vi "DMM Control.vi"(8 "error in (no error)":errorcluster, 10 "JSONCluster":T1 {"DMMVoltageFaultUpperLimit" format="%#_6p"}, 11 "IVI Refnum in":refnum<k15>) -> (0 "error out":errorcluster, 3 "IVI Refnum out":refnum<k15>)   [LabVIEW 2019, in "SupportVIs.lvlib"]
uses:
  SupportVIs.lvlib
  JSONCluster.ctl
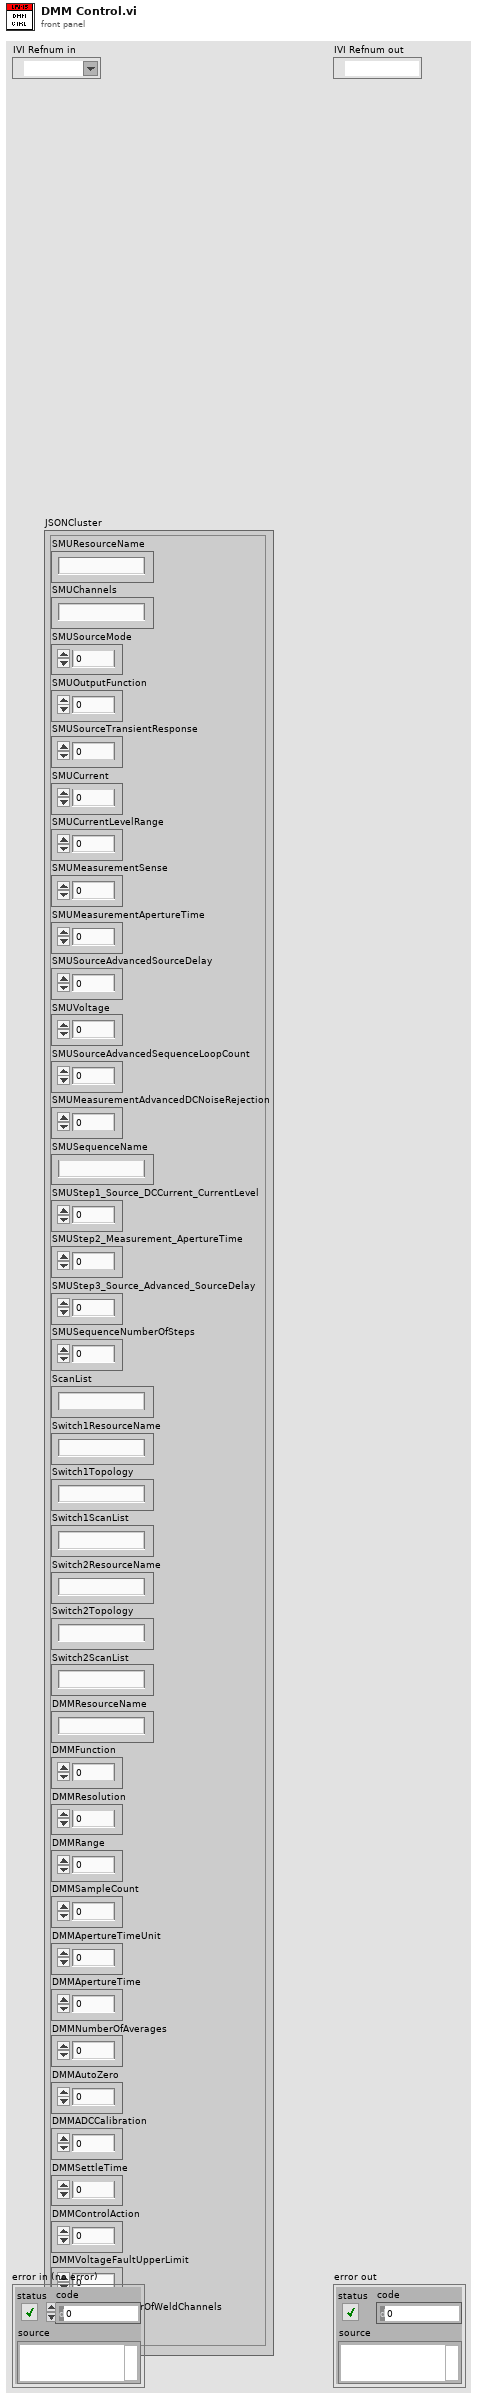
[diagram p1: front panel]
types:
  T1 = typedef "JSONCluster.ctl" = cluster{"SMUResourceName":string, "SMUChannels":string, "SMUSourceMode":i32, "SMUOutputFunction":i32, "SMUSourceTransientResponse":i32, "SMUCurrent":dbl, "SMUCurrentLevelRange":dbl, "SMUMeasurementSense":i32, "SMUMeasurementApertureTime":dbl, "SMUSourceAdvancedSourceDelay":dbl, "SMUVoltage":dbl, "SMUSourceAdvancedSequenceLoopCount":i32, "SMUMeasurementAdvancedDCNoiseRejection":i32, "SMUSequenceName":string, "SMUStep1_Source_DCCurrent_CurrentLevel":i32, "SMUStep2_Measurement_ApertureTime":i32, "SMUStep3_Source_Advanced_SourceDelay":i32, "SMUSequenceNumberOfSteps":i32, "ScanList":string, "Switch1ResourceName":string, "Switch1Topology":string, "Switch1ScanList":string, "Switch2ResourceName":string, "Switch2Topology":string, "Switch2ScanList":string, "DMMResourceName":string, "DMMFunction":i32, "DMMResolution":dbl, "DMMRange":dbl, "DMMSampleCount":i32, "DMMApertureTimeUnit":i32, "DMMApertureTime":dbl, "DMMNumberOfAverages":i32, "DMMAutoZero":i32, "DMMADCCalibration":i32, "DMMSettleTime":dbl, "DMMControlAction":i32, "DMMVoltageFaultUpperLimit":dbl, "ApplicationNumberOfWeldChannels":i32}
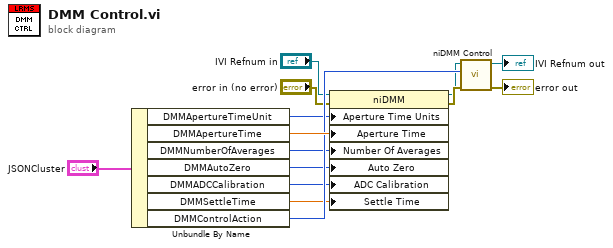
[diagram p0: block diagram]
diagram:
  n1 = Unbundle By Name("JSONCluster") -> ("DMMApertureTimeUnit"=w8:i32, "DMMApertureTime"=w13:dbl, "DMMNumberOfAverages"=w9:i32, "DMMAutoZero"=w1:i32, "DMMADCCalibration"=w10:i32, "DMMSettleTime"=w11:dbl, "DMMControlAction"=w12:i32)
  n2 = property class="niDMM"(reference="IVI Refnum in", error in="error in (no error)", "Aperture Time Units"=w8, "Aperture Time"=w13, "Number Of Averages"=w9, "Auto Zero"=w1, "ADC Calibration"=w10, "Settle Time"=w11) -> (reference out=w6:refnum<k15>, error out=w7:errorcluster)
  n3 = call <instrlib>:"niDMM Control.vi"("error in (no error)"=w7, "Control Action"=w12, "instrument handle"=w6) -> ("error out"=→"error out":errorcluster, "instrument handle out"=→"IVI Refnum out":refnum<k15>)  [unwired: 7 in]
